vi "Run Plugin.vi"(7 "Configuration Entry":string, 8 "error in (no error)":errorcluster, 11 "Configuration Parameters":string[](array[string])) -> (0 "error out":errorcluster, 2 "Logic Entry":T1, 3 "Configuration Entry":T1)   [LabVIEW 2021, in "Python Orchestration.lvlib"]
uses:
  Python Orchestration.lvlib
  Typedef/Scripted Line.ctl
  CIFCore/Common/Typedef/Errors.ctl
  <vilib>/CIF Foundation/CIF Utilities/Errors/Append Error Location.vi
  CIFCore/Common/CIFCoreCommon.lvlib
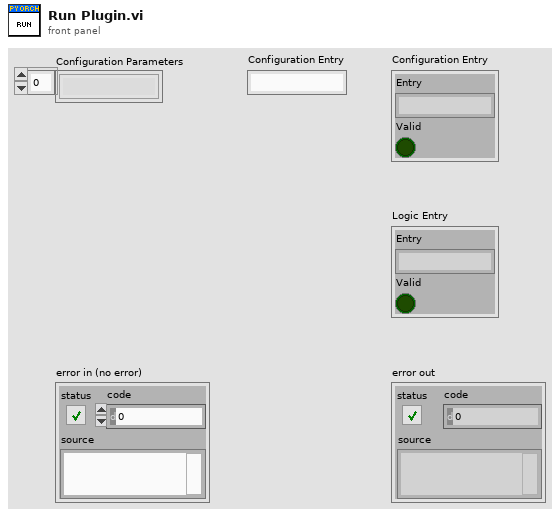
[diagram p1: front panel]
types:
  T1 = typedef "Python Orchestration.lvlib/Scripted Line.ctl" = cluster{"Entry":string, "Valid":bool}
  T2 = typedef "CIFCoreCommon.lvlib/Errors.ctl" = enum16{"Invalid Clock ID", "Long Sleep", "gRPC Server Not Found", "Config Parse", "Timestamp Wrap", "Delayed Execution", "Duplicate Channel", "Missing Channel", "Incorrect Type", "Flatten Error", "Unflatten Data", "Unique Name", "Plugin Not Found", "Plugin Type Not Found", "Plugin Version Not Found", "Manager Not Found", "Numerical Issue", "Time Jump", "Clock ID Match", "Channel Length", "Plugin Connection", "gRPC Server Connection", "PPL Name Match", "Build", "Config Log Parse", "Plugin Load", "UI Subpanel Load", "Python Name", "Invalid Name"}
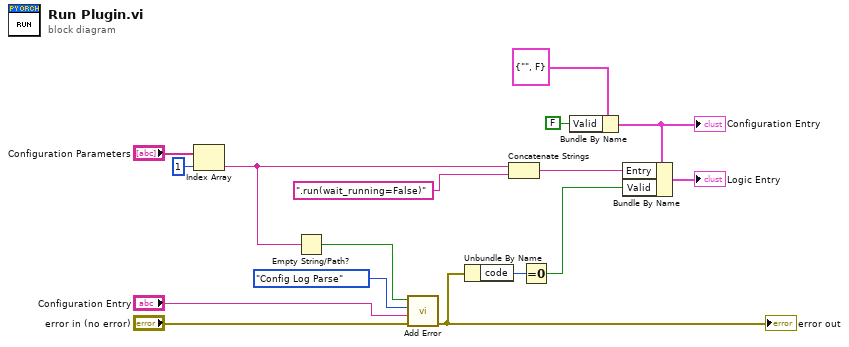
[diagram p0: block diagram]
diagram:
  n1 = Index Array(array="Configuration Parameters", index=1) -> (element=w8:string)
  n2 = Empty String/Path?(string/path=w8) -> (empty?=w1:bool)
  n3 = call "Add Error.vi"("error in (no error)"="error in (no error)", "String to Append"="Configuration Entry", "Error"=Errors."Config Log Parse", "Insert Error"=w1) -> ("error out"=w4:errorcluster)  [unwired: 7 in]
  "error out" <- w4
  n4 = Unbundle By Name(w4) -> ("code"=w16:i32)
  n5 = Concatenate Strings(w8, ".run(wait_running=False)" ("string")) -> (w11:string)
  n6 = Equal To 0?(x=w16) -> (x = 0?=w15:bool)
  n7 = Bundle By Name(cluster=T1 {"Entry"="", "Valid"=FALSE} ("Logic Entry"), "Valid"=FALSE) -> (w7:T1)
  "Configuration Entry" <- w7
  n8 = Bundle By Name(cluster=w7, "Entry"=w11, "Valid"=w15) -> (→"Logic Entry":T1)
